vi "Spin pumping.vi"() -> ()   [LabVIEW 2019]
uses:
  <vilib>/Utility/file.llb/Write Delimited Spreadsheet (DBL).vi
panel:
  in  "Sample Name":string
  in  "Table Control":string[][](table)
  out "Current Measurement Phase":cluster{dbl[], dbl[]}(graph)
  out "Current Measurement Amplitude":cluster{dbl[], dbl[]}(graph)
  out "Last Measurement Phase":cluster{dbl[], dbl[]}(graph)
  out "Last Measurement Amplitude":cluster{dbl[], dbl[]}(graph)
  in  "SR830 GPIB Addr":dbl
  in  "AM Depth (%)":dbl
  in  "AM Freq (Hz)":dbl
  in  "# of pt":dbl
  in  "Kepco Max I":dbl
  in  "Kepco GPIB Addr":dbl
  in  "SMB 100a GPIB Addr":dbl
  in  "Model 7010 GPIB Addr":dbl
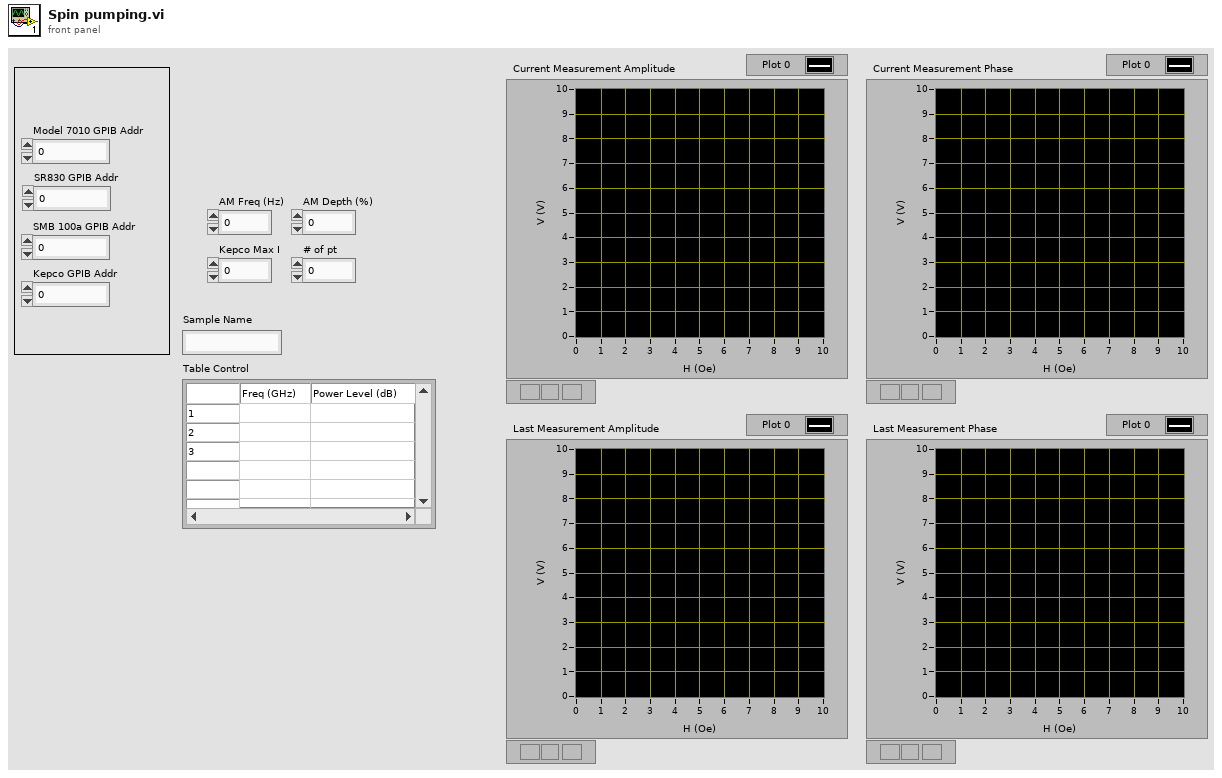
[diagram p1: front panel]
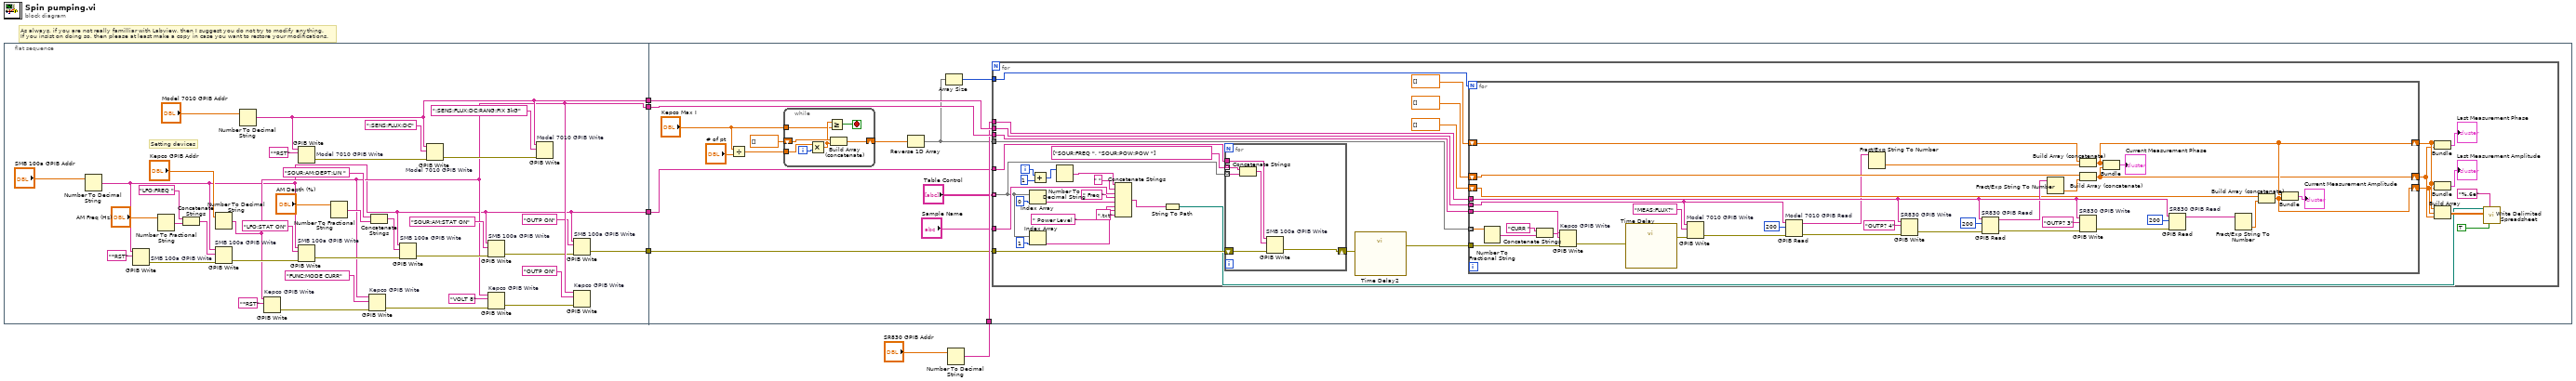
[diagram p0: block diagram]
diagram:
  # "As always, if you are not really familliar with Labview, then I suggest you do not try to modify anything.\nIf you insist on doing so, then please at least make a copy in case you want to restore your modifications."
  n1 = flat-sequence {
    tunnel: [w12] -> w5
    tunnel: [w11] -> w6
    tunnel: [w8] -> w2
    tunnel: [w7] -> w1
    tunnel: w3 -> [w50]
    tunnel: w6 -> [w52]
    tunnel: w5 -> [w51]
    tunnel: w2 -> [w45]
    tunnel: w1 -> [w44]
    frame #0 {
      # "Setting devices"
      n2 = Number To Decimal String(number="SMB 100a GPIB Addr") -> (decimal integer string=w8:string)  [unwired: 1 in]
      n3 = GPIB Write "SMB 100a GPIB Write"(0:w8, 1:"*RST" ("data")) -> (6:w29:errorcluster)  [unwired: 3 in, 1 out]
      n4 = Number To Fractional String(number="AM Freq (Hz)") -> (F-format string=w32:string)  [unwired: 3 in]
      n5 = Concatenate Strings("LFO:FREQ " ("string"), w32) -> (w30:string)
      n6 = Number To Decimal String(number="Kepco GPIB Addr") -> (decimal integer string=w11:string)  [unwired: 1 in]
      n7 = GPIB Write "SMB 100a GPIB Write"(0:w8, 1:w30, 3:w29) -> (6:w28:errorcluster)  [unwired: 2 in, 1 out]
      n8 = Number To Decimal String(number="Model 7010 GPIB Addr") -> (decimal integer string=w12:string)  [unwired: 1 in]
      n9 = GPIB Write "Kepco GPIB Write"(0:w11, 1:"*RST" ("data")) -> (6:w39:errorcluster)  [unwired: 3 in, 1 out]
      n10 = GPIB Write "Model 7010 GPIB Write"(0:w12, 1:"*RST" ("data")) -> (6:w19:errorcluster)  [unwired: 3 in, 1 out]
      n11 = GPIB Write "SMB 100a GPIB Write"(0:w8, 1:"LFO:STAT ON" ("data"), 3:w28) -> (6:w25:errorcluster)  [unwired: 2 in, 1 out]
      n12 = Number To Fractional String(number="AM Depth (%)") -> (F-format string=w24:string)  [unwired: 3 in]
      n13 = GPIB Write "Kepco GPIB Write"(0:w11, 1:"FUNC:MODE CURR" ("data"), 3:w39) -> (6:w37:errorcluster)  [unwired: 2 in, 1 out]
      n14 = Concatenate Strings("SOUR:AM:DEPT:LIN " ("string"), w24) -> (w23:string)
      n15 = GPIB Write "SMB 100a GPIB Write"(0:w8, 1:w23, 3:w25) -> (6:w21:errorcluster)  [unwired: 2 in, 1 out]
      n16 = GPIB Write "Model 7010 GPIB Write"(0:w12, 1:":SENS:FLUX:DC" ("data"), 3:w19) -> (6:w17:errorcluster)  [unwired: 2 in, 1 out]
      n17 = GPIB Write "SMB 100a GPIB Write"(0:w8, 1:"SOUR:AM:STAT ON" ("data"), 3:w21) -> (6:w10:errorcluster)  [unwired: 2 in, 1 out]
      n18 = GPIB Write "Kepco GPIB Write"(0:w11, 1:"VOLT 8" ("data"), 3:w37) -> (6:w35:errorcluster)  [unwired: 2 in, 1 out]
      n19 = GPIB Write "Model 7010 GPIB Write"(0:w12, 1:":SENS:FLUX:DC:RANG:FIX 3kG" ("data"), 3:w17) -> ()  [unwired: 2 in, 2 out]
      n20 = GPIB Write "SMB 100a GPIB Write"(0:w8, 1:"OUTP ON" ("data"), 3:w10) -> (6:w7:errorcluster)  [unwired: 2 in, 1 out]
      n21 = GPIB Write "Kepco GPIB Write"(0:w11, 1:"OUTP ON" ("data"), 3:w35) -> ()  [unwired: 2 in, 2 out]
    }
    frame #1 {
      n22 = Divide(x="Kepco Max I", y="# of pt") -> (x/y=w55:dbl)
      n23 = while {
        tunnel: w55 -> [w140]
        shift-right: [w139] -> w53
        shift-left: dbl[] [] -> [w138]
        tunnel: "Kepco Max I" -> [w135]
        i -> [w141]
        stop <- w137 stop-if-true
        n24 = Multiply(x=w140, y=w141) -> (x*y=w136:dbl)
        n25 = Greater Or Equal?(x=w136, y=w135) -> (x >= y?=w137:bool)
        n26 = Build Array (concatenate)(w138, w136) -> (w139:dbl[])
      }
      n27 = Reverse 1D Array(array=w53) -> (reversed array=w49:dbl[])
      n28 = Array Size(array=w49) -> (size(s)=w48:i32)
      n29 = for {
        tunnel: w52 -> [w91]
        tunnel: w51 -> [w90]
        tunnel: w50 -> [w89]
        tunnel: w49 -> [w80]
        tunnel: w48 -> [w79]
        tunnel: "Table Control" -> [w63] mode=indexing
        tunnel: w45 -> [w76]
        tunnel: w44 -> [w75]
        tunnel: "Sample Name" -> [w67]
        i -> [w72]
        n30 = Index Array(array=w63, index=0) -> (element=w65:string)
        n31 = Index Array(array=w63, index=1) -> (element=w60:string)
        n32 = Add(x=w72, y=1) -> (x+y=w70:i32)
        n33 = Number To Decimal String(number=w70) -> (decimal integer string=w69:string)  [unwired: 1 in]
        n34 = Concatenate Strings(w69, " " ("string"), w67, " Freq " ("string"), w65, " Power Level " ("string"), w60, ".txt" ("string")) -> (w58:string)
        n35 = String To Path(string=w58) -> (path=w57:path)
        n36 = for {
          tunnel: w63 -> [w98] mode=indexing
          tunnel: string[] ["SOUR:FREQ ", "SOUR:POW:POW "] -> [w99] mode=indexing
          tunnel: w76 -> [w96]
          shift-right: [w95] -> w74
          shift-left: w75 -> [w94]
          n37 = Concatenate Strings(w99, w98) -> (w97:string)
          n38 = GPIB Write "SMB 100a GPIB Write"(0:w96, 1:w97, 3:w94) -> (6:w95:errorcluster)  [unwired: 2 in, 1 out]
        }
        n39 = call "Time Delay2"("error in (no error)"=w74) -> ("error out"=w73:errorcluster)  [unwired: 10 in]
        n40 = for {
          N: w79 -> [_]
          tunnel: w80 -> [w133] mode=indexing
          tunnel: w91 -> [w130]
          tunnel: w90 -> [w114]
          tunnel: w89 -> [w122]
          shift-right: [w107] -> w82
          shift-left: dbl[] [] -> [w119]
          shift-right: [w108] -> w83
          shift-left: dbl[] [] -> [w116]
          shift-right: [w109] -> w85
          shift-left: dbl[] [] -> [w110]
          tunnel: w73 -> [w100]
          n41 = Number To Fractional String(number=w133) -> (F-format string=w132:string)  [unwired: 3 in]
          n42 = Concatenate Strings("CURR ", w132) -> (w131:string)
          n43 = GPIB Write "Kepco GPIB Write"(0:w130, 1:w131, 3:w100) -> (6:w129:errorcluster)  [unwired: 2 in, 1 out]
          n44 = call "Time Delay"("error in (no error)"=w129) -> ("error out"=w128:errorcluster)  [unwired: 10 in]
          n45 = GPIB Write "Model 7010 GPIB Write"(0:w114, 1:"MEAS:FLUX?" ("data"), 3:w128) -> (6:w113:errorcluster)  [unwired: 2 in, 1 out]
          n46 = GPIB Read "Model 7010 GPIB Read"(0:w114, 1:200 ("byte count"), 3:w113) -> (5:w111:string, 7:w112:errorcluster)  [unwired: 2 in, 1 out]
          n47 = Fract/Exp String To Number(string=w111) -> (number=w115:dbl)  [unwired: 3 in, 1 out]
          n48 = GPIB Write "SR830 GPIB Write"(0:w122, 1:"OUTP? 4" ("data"), 3:w112) -> (6:w125:errorcluster)  [unwired: 2 in, 1 out]
          n49 = GPIB Read "SR830 GPIB Read"(0:w122, 1:200 ("byte count"), 3:w125) -> (5:w121:string, 7:w124:errorcluster)  [unwired: 2 in, 1 out]
          n50 = Fract/Exp String To Number(string=w121) -> (number=w120:dbl)  [unwired: 3 in, 1 out]
          n51 = Build Array (concatenate)(w110, w115) -> (w109:dbl[])
          n52 = Build Array (concatenate)(w119, w120) -> (w107:dbl[])
          n53 = GPIB Write "SR830 GPIB Write"(0:w122, 1:"OUTP? 3" ("data"), 3:w124) -> (6:w123:errorcluster)  [unwired: 2 in, 1 out]
          n54 = Bundle(w109, w107) -> (→"Current Measurement Phase":cluster{dbl[], dbl[]})  [unwired: 1 in]
          n55 = GPIB Read "SR830 GPIB Read"(0:w122, 1:200 ("byte count"), 3:w123) -> (5:w117:string)  [unwired: 2 in, 2 out]
          n56 = Fract/Exp String To Number(string=w117) -> (number=w118:dbl)  [unwired: 3 in, 1 out]
          n57 = Build Array (concatenate)(w116, w118) -> (w108:dbl[])
          n58 = Bundle(w109, w108) -> (→"Current Measurement Amplitude":cluster{dbl[], dbl[]})  [unwired: 1 in]
        }
        n59 = Bundle(w85, w82) -> (→"Last Measurement Phase":cluster{dbl[], dbl[]})  [unwired: 1 in]
        n60 = Bundle(w85, w83) -> (→"Last Measurement Amplitude":cluster{dbl[], dbl[]})  [unwired: 1 in]
        n61 = Build Array(w85, w83, w82) -> (w84:dbl[][])
        n62 = call-poly <vilib>:"Write Delimited Spreadsheet.vi"("file path (dialog if empty)"=w57, "format (%.3f)"="%.6e", "2D data"=w84, "transpose? (no:F)"=TRUE) -> ()  [unwired: 10 in, 2 out]
      }
    }
  }
  n63 = Number To Decimal String(number="SR830 GPIB Addr") -> (decimal integer string=w3:string)  [unwired: 1 in]
